vi "intraloop FIFO test.vi"() -> ()   [LabVIEW 2018]
panel:
  out "read elements":u32
  out "write elements":u32
  out "message received":T1(ring)
  out "reading":bool
  in  "quit":bool
  in  "send":bool
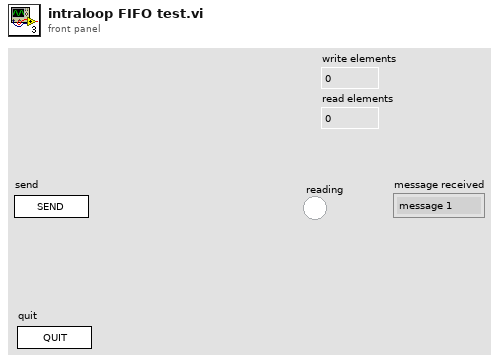
[diagram p1: front panel]
types:
  T1 = enum16{"message 1", "message 2", "message X", "message N"}
  T2 = enum16{"message 1", "message 2", "message X", "message N"}[]
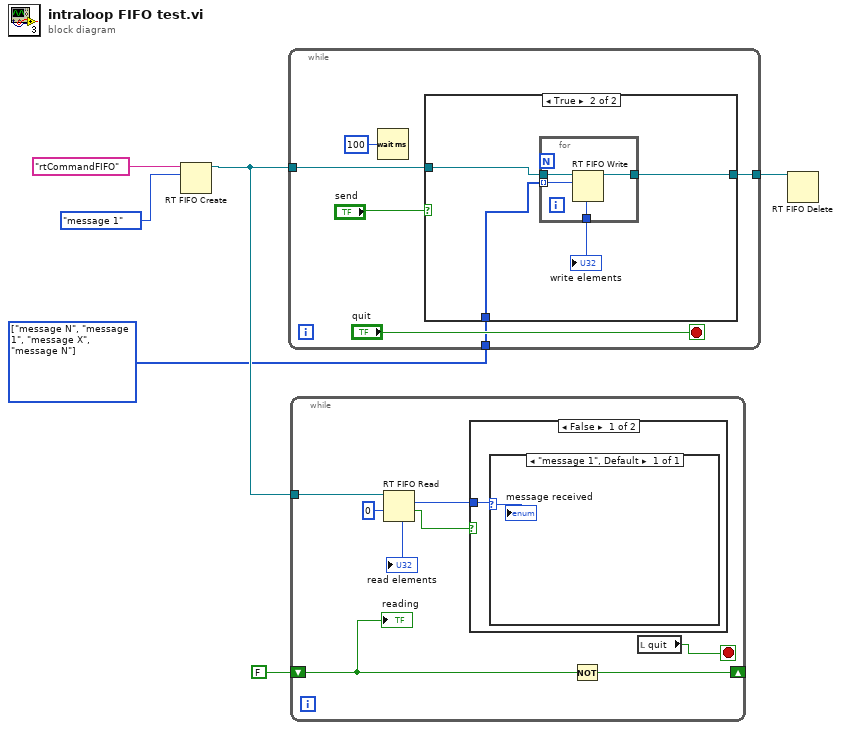
[diagram p0: block diagram]
diagram:
  w2 = T2 [enum."message N", enum."message 1", enum."message X", enum."message N"] items=["message 1", "message 2", "message X", "message N"] ("message enum 2")
  n1 = RT FIFO Create(0:"rtCommandFIFO" ("name (unnamed)"), 1:T1."message 1" ("message enum 2")) -> (8:w5:refnum<k33>)  [unwired: 6 in, 2 out]
  n2 = while {
    tunnel: w5 -> [w9]
    tunnel: w2 -> [w8]
    tunnel: [w7] -> w1
    stop <- "quit" stop-if-true
    n3 = Wait (ms)(milliseconds to wait=u32 100) -> ()  [unwired: 1 out]
    n4 = case shown="True" "send" {
      tunnel: w9 -> [w13 w17]
      tunnel: w8 -> [_ w15]
      tunnel: [w13 w14] -> w7
      frame False {
      }
      frame True {
        n5 = for {
          tunnel: w17 -> [w21]
          tunnel: [w20] -> w16
          tunnel: w15 -> [w19] mode=indexing
          tunnel: [w18] -> w14
          n6 = RT FIFO Write(0:w21, 1:w19) -> (7:w20:u32, 8:w18:refnum<k33>)  [unwired: 3 in, 2 out]
        }
        "write elements" <- w16
      }
    }
  }
  n7 = while {
    tunnel: w5 -> [w28]
    shift-right: [w23] -> _
    shift-left: FALSE -> [w22]
    stop <- w29 stop-if-true
    n8 = RT FIFO Read(0:w28, 2:0 ("timeout in ms (0)")) -> (7:→"read elements":u32, 9:w27:T1, 10:w25:bool)  [unwired: 2 in, 2 out]
    n9 = case shown="False" w25 {
      tunnel: w27 -> [w30 _]
      frame False {
        n10 = case shown="\"message 1\", Default" w30 {
          selector: w30 -> [w31]
          frame "message 1", Default {
            "message received" <- w31
          }
        }
      }
      frame True {
      }
    }
    n11 = Not(x=w22) -> (.not. x?=w23:bool)
    n12 = local read "quit"() -> (w29:bool)
    "reading" <- w22
  }
  n13 = RT FIFO Delete(0:w1) -> ()  [unwired: 2 in, 1 out]
